vi "Write Time Scale.vi"(8 "error in (no error)":errorcluster, 10 "Time Scale [ms]":u32, 11 "Worker In":refnum<class "Worker.lvclass">) -> (0 "error out":errorcluster, 3 "Worker Out":refnum<class "Worker.lvclass">)   [LabVIEW 2020, in "Worker.lvclass"]
uses:
  Worker/Worker.lvclass
  Worker/Worker.lvclass/Worker.ctl
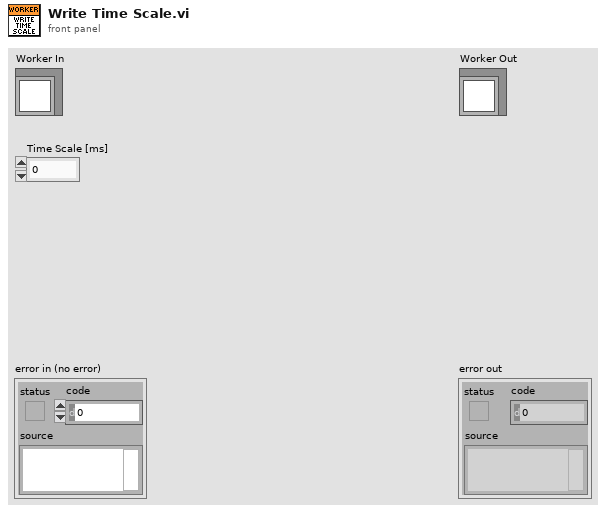
[diagram p1: front panel]
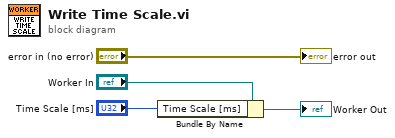
[diagram p0: block diagram]
diagram:
  n1 = Bundle By Name(cluster="Worker In", "Time Scale [ms]"="Time Scale [ms]") -> (→"Worker Out":refnum<class "Worker.lvclass">)
  "error out" <- "error in (no error)"
